vi "Tell Self.vi"(4 "Priority":bool, 7 "Actor in":refnum<class "Actor.lvclass">, 9 "Parent Stopped":bool, 10 "Safe Stop":bool=TRUE) -> (0 "Error out":errorcluster)   [LabVIEW 2025, in "jettl.lvlib" / "Stop jettl Msg.lvlib"]
uses:
  Stop jettl Msg.lvlib
  Msg Input/Msg Input.lvclass
  Stop Msg/Stop Msg/Stop Msg.lvclass
  C:/git/jettl/src/jettl/jettl/Stop jettl Msg/Stop Msg/Stop Msg/Stop Msg.lvclass
  C:/git/jettl/src/jettl/jettl/Msg/Msg.lvclass
  jettl.lvlib
  Actor/Actor.lvclass
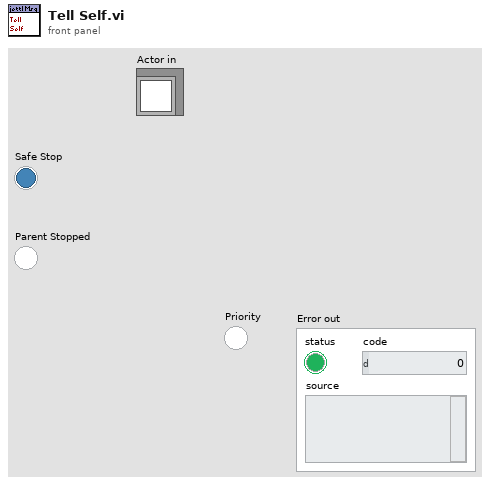
[diagram p1: front panel]
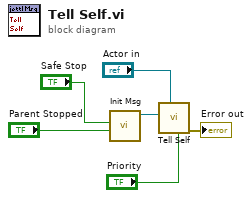
[diagram p0: block diagram]
diagram:
  n1 = call "Init Msg.vi"(9:"Parent Stopped", "Msg Input"="Safe Stop") -> ("Stop Msg out"=w3:refnum<class "Stop Msg.lvclass">)  [unwired: 9 in]
  n2 = call "Tell Self.vi"("Priority"="Priority", "Actor in"="Actor in", "Msg"=w3) -> ("Error out"=→"Error out":errorcluster)  [unwired: 8 in]
